vi "[FPGA] True RMS Power Quality Analyzer Multichannel 00.vi"(0 "V [V]":sgl, 1 "I [A]":sgl, 3 "LTYPE":sgl=1.0, 4 "Channel #":u32, 5 "dt (s)":sgl=3e-05, 7 "reinitialize? (F)":bool, 9 "Debounce (iterations)":i32=5) -> (15 "Power Analysis":T1)   [LabVIEW 2015]
uses:
  IP Cores/IP Cores - LabVIEW FPGA/Floating Point/Polymorphic subVIs/Multiply 00.vi
  IP Cores/IP Cores - LabVIEW FPGA/Floating Point/Polymorphic subVIs/Divide 00.vi
  IP Cores/IP Cores - LabVIEW FPGA/Floating Point/Polymorphic subVIs/Square Root 00.vi
  IP Cores/IP Cores - LabVIEW FPGA/Floating Point/Polymorphic subVIs/Subtract 00.vi
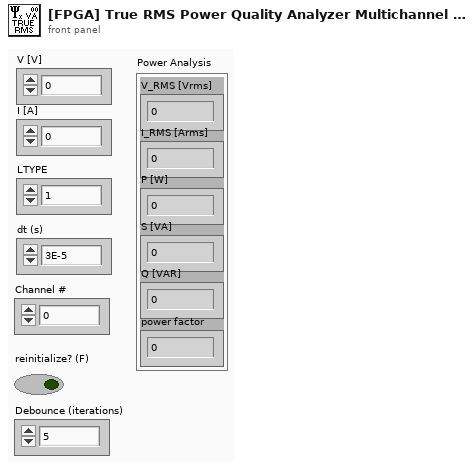
[diagram p1: front panel]
types:
  T1 = cluster{"V_RMS [Vrms] ":sgl, "I_RMS [Arms]":sgl, "P [W]":sgl, "S [VA]":sgl, "Q [VAR]":sgl, "power factor":sgl}
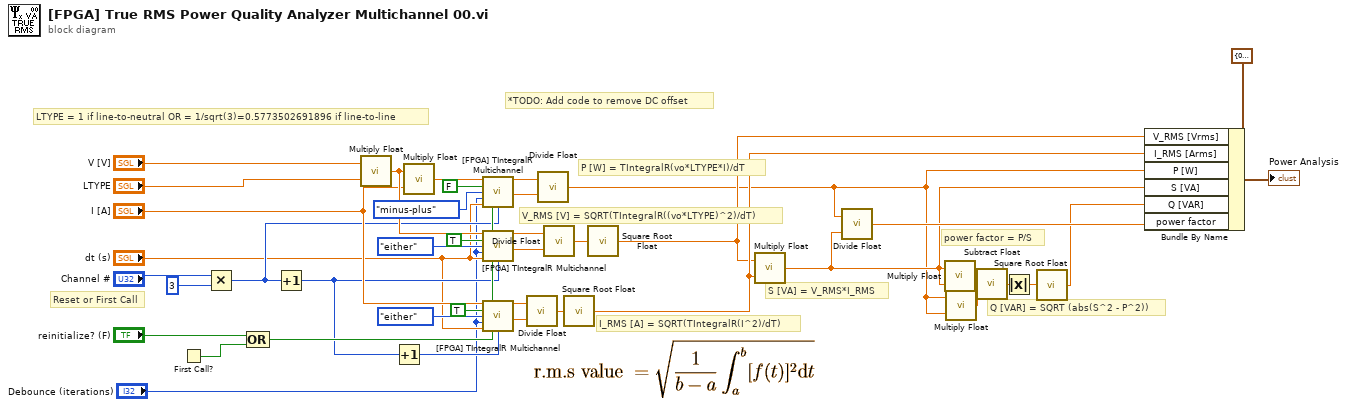
[diagram p0: block diagram]
diagram:
  # "*TODO: Add code to remove DC offset"
  # "LTYPE = 1 if line-to-neutral OR = 1/sqrt(3)=0.5773502691896 if line-to-line"
  # "power factor = P/S"
  # "Q [VAR] = SQRT (abs(S^2 - P^2))"
  # "S [VA] = V_RMS*I_RMS"
  # "I_RMS [A] = SQRT(TIntegralR(I^2)/dT)"
  # "P [W] = TIntegralR(vo*LTYPE*I)/dT"
  # "V_RMS [V] = SQRT(TIntegralR((vo*LTYPE)^2)/dT)"
  # "Reset or First Call"
  n1 = First Call?() -> (First Call?: T/F=w40:bool)
  n2 = Multiply(x="Channel #", y=u32 3) -> (x*y=w15:u32)
  n3 = Compound Arithmetic op=OR("reinitialize? (F)", w40) -> (w23:bool)
  n4 = Increment(x=w15) -> (x+1=w14:u32)
  n5 = call-poly "Multiply Float.vi"("y"="LTYPE", "x"="V [V]") -> ("x*y"=w29:sgl)
  n6 = Increment(x=w14) -> (x+1=w13:u32)
  n7 = call-poly "Multiply Float.vi"("y"="I [A]", "x"=w29) -> ("x*y"=w33:sgl)
  n8 = call "[FPGA] TIntegralR Multichannel.vi"("x{k}"=w33, "reset"=w23, "x^2?"=FALSE, "zero cross direction"=enum8{"either", "minus-plus", "plus-minus"}."minus-plus", "Debounce (iterations)"="Debounce (iterations)", "dt (s)"="dt (s)", "Channel #"=w15) -> ("TIntegralR(x{k})"=w32:sgl, "dT [s]"=w27:sgl)  [unwired: 7 in]
  n9 = call "[FPGA] TIntegralR Multichannel.vi"("x{k}"=w29, "reset"=w23, "x^2?"=TRUE, "zero cross direction"=enum8{"either", "minus-plus", "plus-minus"}."either", "Debounce (iterations)"="Debounce (iterations)", "dt (s)"="dt (s)", "Channel #"=w14) -> ("TIntegralR(x{k})"=w19:sgl, "dT [s]"=w1:sgl)  [unwired: 7 in]
  n10 = call "[FPGA] TIntegralR Multichannel.vi"("x{k}"="I [A]", "reset"=w23, "x^2?"=TRUE, "zero cross direction"=enum8{"either", "minus-plus", "plus-minus"}."either", "Debounce (iterations)"="Debounce (iterations)", "dt (s)"="dt (s)", "Channel #"=w13) -> ("TIntegralR(x{k})"=w18:sgl, "dT [s]"=w31:sgl)  [unwired: 7 in]
  n11 = call-poly "Divide Float.vi"("y"=w31, "x"=w18) -> ("x/y"=w16:sgl)
  n12 = call-poly "Divide Float.vi"("y"=w27, "x"=w32) -> ("x/y"=w3:sgl)
  n13 = call-poly "Divide Float.vi"("y"=w1, "x"=w19) -> ("x/y"=w17:sgl)
  n14 = call-poly "Square Root Float.vi"("x"=w16) -> ("sqrt(x)"=w6:sgl)
  n15 = call-poly "Square Root Float.vi"("x"=w17) -> ("sqrt(x)"=w5:sgl)
  n16 = call-poly "Multiply Float.vi"("y"=w6, "x"=w5) -> ("x*y"=w7:sgl)
  n17 = call-poly "Divide Float.vi"("y"=w7, "x"=w3) -> ("x/y"=w9:sgl)
  n18 = call-poly "Multiply Float.vi"("y"=w7, "x"=w7) -> ("x*y"=w36:sgl)
  n19 = call-poly "Multiply Float.vi"("y"=w3, "x"=w3) -> ("x*y"=w35:sgl)
  n20 = call-poly "Subtract Float.vi"("y"=w35, "x"=w36) -> ("x*y"=w30:sgl)
  n21 = Absolute Value(x=w30) -> (abs(x)=w34:sgl)
  n22 = call-poly "Square Root Float.vi"("x"=w34) -> ("sqrt(x)"=w8:sgl)
  n23 = Bundle By Name(cluster=T1 {"V_RMS [Vrms] "=0.0, "I_RMS [Arms]"=0.0, "P [W]"=0.0, "S [VA]"=0.0, "Q [VAR]"=0.0, "power factor"=0.0} ("Power Analysis"), "V_RMS [Vrms]"=w5, "I_RMS [Arms]"=w6, "P [W]"=w3, "S [VA]"=w7, "Q [VAR]"=w8, "power factor"=w9) -> (→"Power Analysis":T1)
